vi "IP_POWER1_Off_WebSwitch_Control.vi"() -> ()   [LabVIEW 2011]
doc: "Example of using standard HTTP protocol for recieving a web site (the HTML source)\n\n\nThis example uses the GET command. For general information about the HTTP protocol and other commands go to\nhttp://www.w3.org/Protocols\n\n\nBjornar Svingen\nbjornar.svingen@sintef.no bjornar.svingen@ktv.no"
uses:
  Instance           2 38Saved   IP_POWER_Off_WebSwitch_Control .vi
  Instance           6 38Saved   IP_POWER_Off_WebSwitch_Control .vi
panel:
  out "Begin Time":u32
  out "SW OU2 ON/OFF":bool=TRUE
  out "SW OU1 ON/OFF":bool=TRUE
  out "standard output":string
  out "PING WEBSW IP CMD":string
  out "code 2":i32
  out "Setup WEBSW IP CMD":string
  out "code":i32
  out "WEBSW_SN":string
  out "WEBSW_IP":string
  out "text":string
  out "Setup Status":bool
  out "result string":string
  out "Device SW State":bool[](array[boolean])
  out "Seach the specific string":string[](array[string])
  out "OUT CMD":string[](array[string])
  out "OUT2 CMD":string="/state.xml?relay2State=1"
  out "OUT1 CMD":string="/state.xml?relay1State=1"
  out "HTML source":string
  # "小心它是110V"
  # "2014-10-8"
  # "Web Switch Control"
  # "POWER1 off"
  # "PowerOff"
  # "Command\nhttp://Device IP/state.xml?relay1State=0\nhttp://Device IP/state.xml?relay1State=1\nhttp://Device IP/state.xml?relay2State=0\nhttp://Device IP/state.xml?relay2State=1"
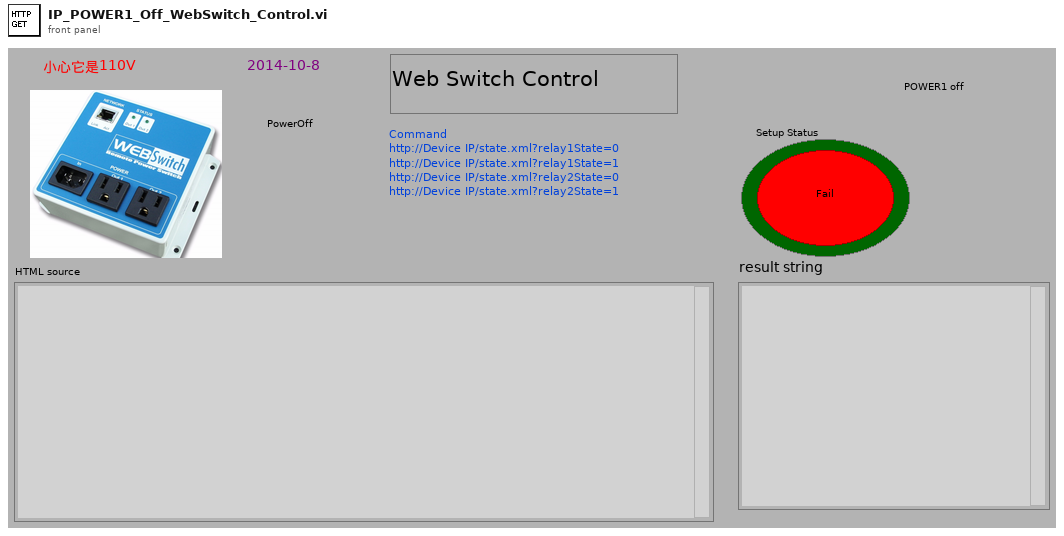
[diagram p1: front panel]
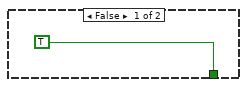
[diagram p5: hidden frame]
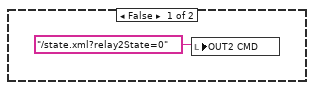
[diagram p7: hidden frame]
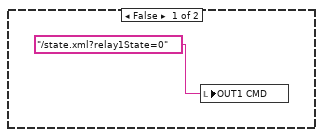
[diagram p8: hidden frame]
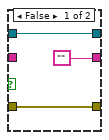
[diagram p9: hidden frame]
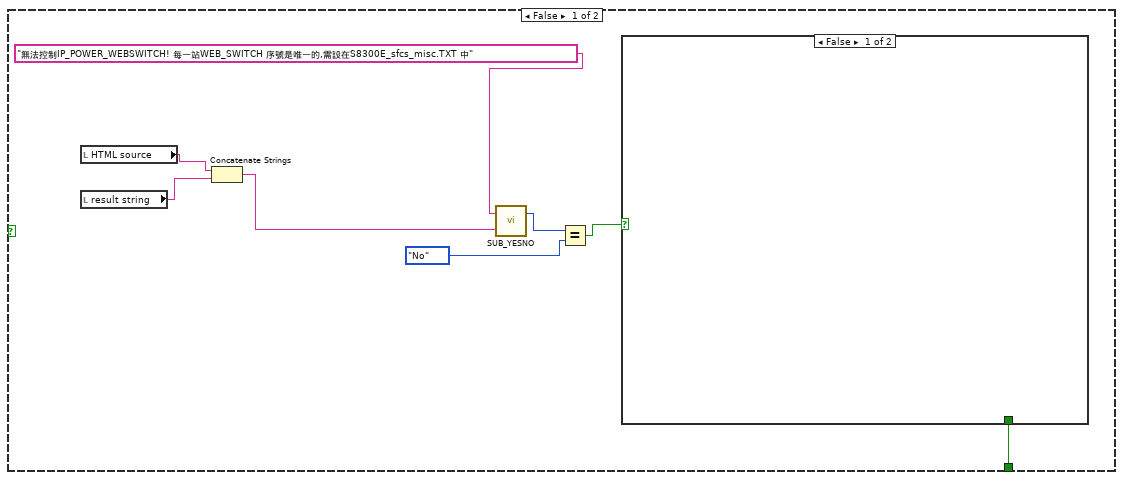
[diagram p10: hidden frame]
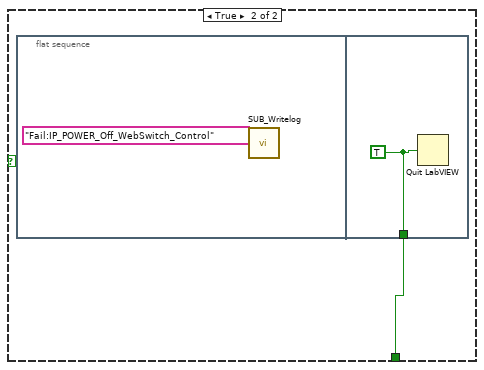
[diagram p11: hidden frame]
diagram:
  n1 = while {
    i -> [w1]
    stop <- w2 stop-if-true
    n2 = flat-sequence {
      tunnel: w1 -> [w4]
      tunnel: [w127] -> w2
      frame #0 {
        n3 = Equal To 0?(x=w4) -> (x = 0?=w3:bool)
        n4 = case shown="True" w3 {
          frame False {
          }
          frame True {
            n5 = Tick Count (ms)() -> (millisecond timer value=→"Begin Time":u32)
          }
        }
      }
      frame #1 {
        w8 = ""
        # "To assign the temporary IP address...\n1. Make sure  WebSwitch TM  and the configuration computer are connected to the same physical\nnetwork.  This will not work through routers or gateways.\n2. Assign the address as follows...\nWindows:\nOpen a Command Prompt (on Windows XP, select START, then RUN, then type “cmd”).\nType...\narp -s {new IP address} {serial number of  WebSwitch TM  }Revision 1.01                           WebSwitch TM    Users Manual\nXytronix Research & Design, Inc.                  page 6\nNote:   IP address format is: xxx.xxx.xxx.xxx\nSerial number format is: ss-ss-ss-ss-ss-ss\nFor example, to set a WebSwitch TM  device (with serial number 00-0C-C8-01-00-01 )  to\n10.10.10.40 the following command would be used.\narp -s 10.10.10.40 00-0c-c8-01-00-01"
        n6 = local write "OUT1 CMD"(w8) -> ()
        n7 = local write "OUT2 CMD"(w8) -> ()
        n8 = local write "result string"(w8) -> ()
        "SW OU1 ON/OFF" <- FALSE ("SW OU1 ON/OFF")
        "SW OU2 ON/OFF" <- FALSE ("SW OU2 ON/OFF")
      }
      frame #2 {
        n9 = call "SUB_SearchFile_inFolder.vi"("Search Filename in Folder"="S8300E_sfcs_misc.TXT") -> ("File Existing True/Flase"=w9:bool)  [unwired: 1 in]
        n10 = case shown="False" w9 {
          frame False {
            n11 = flat-sequence {
              frame #0 {
                n12 = call "Display Message to User2"() -> ()  [unwired: 10 in, 2 out]
              }
              frame #1 {
                n13 = call "SUB_Writelog.vi"("Pass/Fail"="Fail:IP_POWER_Off_WebSwitch_Control") -> ()  [unwired: 2 in]
              }
              frame #2 {
                n14 = Quit LabVIEW(quit? (T)=TRUE) -> ()
              }
            }
          }
          frame True {
          }
        }
      }
      frame #3 {
        n15 = call "SUB_Read_specifFile.vi"("name or relative path"="S8300E_sfcs_misc.TXT") -> ("text"=w19:string)  [unwired: 1 in, 1 out]
        "text" <- w19
        n16 = call "SUB_FindSpecificString.vi"("Find this String"="IP_POWER_WEB_SWITCH_IP=", "String data"=w19) -> ("before \"; \" string"=→"WEBSW_IP":string, "Found"=w17:bool)  [unwired: 2 in]
        n17 = call "SUB_FindSpecificString.vi"("Find this String"="IP_POWER_WEB_SWITCH_SN=", "String data"=w19) -> ("before \"; \" string"=→"WEBSW_SN":string, "Found"=w16:bool)  [unwired: 2 in]
        n18 = And(x=w17, y=w16) -> (x .and. y?=w15:bool)
        n19 = case shown="False" w15 {
          frame False {
            n20 = flat-sequence {
              frame #0 {
                n21 = call "Display Message to User"() -> ()  [unwired: 10 in, 2 out]
              }
              frame #1 {
                n22 = call "SUB_Writelog.vi"("Pass/Fail"="Fail:IP_POWER_Off_WebSwitch_Control") -> ()  [unwired: 2 in]
              }
              frame #2 {
                n23 = Quit LabVIEW(quit? (T)=TRUE) -> ()
              }
            }
          }
          frame True {
          }
        }
      }
      frame #4 {
        n24 = local read "WEBSW_IP"() -> (w26:string)
        n25 = local read "WEBSW_SN"() -> (w29:string)
        n26 = Concatenate Strings("ping -l 102 ", w26, "  -n 1") -> (→"PING WEBSW IP CMD":string)
        n27 = Concatenate Strings("arp -S ", w26, "  ", w29) -> (→"Setup WEBSW IP CMD":string)
      }
      frame #5 {
        n28 = while {
          stop <- w33 stop-if-true
          n29 = flat-sequence {
            tunnel: [w39] -> w32
            tunnel: [w48] -> w33
            tunnel: w32 -> [w45]
            frame #0 {
              n30 = Concatenate Strings("arp -d *" ("string"), "\r") -> (w36:string)
              n31 = call "SUB_run_exeFile_Textv2.vi"("exe filename"=w36) -> ()  [unwired: 1 in, 2 out]
            }
            frame #1 {
              (unwired) "CMD /C"
              n32 = local read "Setup WEBSW IP CMD"() -> (w40:string)
              n33 = Concatenate Strings(w40, "\r") -> (w38:string)
              n34 = call "SUB_run_exeFile_Textv2.vi"("exe filename"=w38) -> ("code"=w37:i32)  [unwired: 1 in, 1 out]
              "code" <- w37
              n35 = Not Equal To 0?(x=w37) -> (x != 0?=w39:bool)
            }
            frame #2 {
              (unwired) "CMD /C"
              n36 = local read "PING WEBSW IP CMD"() -> (w53:string)
              n37 = Concatenate Strings(w53, "\r") -> (w43:string)
              n38 = call "SUB_run_exeFile_Textv2.vi"("exe filename"=w43) -> ("code"=→"code 2":i32, "standard output"=w44:string)  [unwired: 1 in]
              "standard output" <- w44
              n39 = call "SUB_FindSpecificString.vi"("Find this String"="Request timed out", "String data"=w44) -> ("Found"=w50:bool)  [unwired: 2 in, 1 out]
              n40 = call "SUB_FindSpecificString.vi"("Find this String"="unreachable", "String data"=w44) -> ("Found"=w49:bool)  [unwired: 2 in, 1 out]
              n41 = Or(x=w50, y=w49) -> (x .or. y?=w47:bool)
              n42 = Or(x=w47, y=w45) -> (x .or. y?=w46:bool)
              n43 = case shown="True" w46 {
                tunnel: w44 -> [_ w59]
                tunnel: [TRUE w56] -> w48
                frame False {
                }
                frame True {
                  # "cc"
                  n44 = call "SUB_YESNO.vi"("Debug View"=w59, "Status"="無法成功Ping WEB Switch ! WEB SW 序號也要設對於文檔S8300E_sfcs_misc.TXT中!") -> ("yes/no"=w58:enum32{"No Selection", "Yes", "No", "None"})  [unwired: 1 in]
                  n45 = Equal?(x=w58, y=enum32{"No Selection", "Yes", "No", "None"}."No") -> (x = y?=w56:bool)
                  n46 = case shown="True" w56 {
                    frame False {
                    }
                    frame True {
                      n47 = flat-sequence {
                        frame #0 {
                          n48 = call "SUB_Writelog.vi"("Pass/Fail"="Fail:IP_POWER_Off_WebSwitch_Control") -> ()  [unwired: 2 in]
                        }
                        frame #1 {
                          n49 = Quit LabVIEW(quit? (T)=TRUE) -> ()
                        }
                      }
                    }
                  }
                }
              }
            }
          }
        }
      }
      frame #6 {
        n50 = local read "SW OU1 ON/OFF"() -> (w64:bool)
        n51 = local read "SW OU2 ON/OFF"() -> (w63:bool)
        n52 = case shown="True" w64 {
          frame False {
            n53 = local write "OUT1 CMD"("/state.xml?relay1State=0") -> ()
          }
          frame True {
            "OUT1 CMD" <- "/state.xml?relay1State=1"
          }
        }
        n54 = case shown="True" w63 {
          frame False {
            n55 = local write "OUT2 CMD"("/state.xml?relay2State=0") -> ()
          }
          frame True {
            "OUT2 CMD" <- "/state.xml?relay2State=1"
          }
        }
      }
      frame #7 {
        n56 = local read "OUT2 CMD"() -> (w76:string)
        n57 = local read "OUT1 CMD"() -> (w77:string)
        n58 = Build Array(FALSE, FALSE) -> (→"Device SW State":bool[])
        n59 = Build Array("relay1state1", "relay2state1") -> (→"Seach the specific string":string[])
        n60 = Build Array(w77, w76) -> (→"OUT CMD":string[])
      }
      frame #8 {
      }
      frame #9 {
        n61 = for {
          N: 1 -> [_]
          i -> [w89]
          # "Compose the header\n(can include lots of things, see www.w3.org/Protodols)"
          # "The GET method is used to recieve a website.\n\nThe header is composed according to the HTTP 1.1 standard"
          # "Close the connection"
          # "If error code=66, meaning the server\nhas transferred all the data and closed\nthe connection, treat this error as no error."
          # "Read the reply\n(from the GET method)\nin 1024 byte blocks\nand stop on any error."
          # "Write the \"header\"\nto the web site"
          # "Open TCP connection at\nspecifyed web site"
          n62 = local read "WEBSW_IP"() -> (w79:string)
          n63 = TCP Open Connection(address=w79, remote port or service name=u16 80 ("remote port")) -> (connection ID=w85:refnum<k5>, error out=w84:errorcluster)  [unwired: 3 in]
          n64 = local read "OUT CMD"() -> (w96:string[])
          n65 = call <vilib>:"Trim Whitespace.vi"("string"=w79) -> ("trimmed string"=w99:string)  [unwired: 1 in]
          n66 = Index Array(array=w96, index=w89) -> (element=w95:string)
          n67 = call <vilib>:"Trim Whitespace.vi"("string"=w95) -> ("trimmed string"=w103:string)  [unwired: 1 in]
          n68 = local read "Seach the specific string"() -> (w94:string[])
          n69 = Concatenate Strings("GET " ("Command"), w103, " HTTP/1.1" ("Command"), "\r\n" ("string"), "Host: " ("Command"), w99, "\r\n\r\n" ("string")) -> (w97:string)
          n70 = TCP Write(connection ID=w85, data in=w97, error in (no error)=w84) -> (connection ID out=w111:refnum<k5>, error out=w110:errorcluster)  [unwired: 1 in, 1 out]
          n71 = while {
            tunnel: w110 -> [w125]
            tunnel: w111 -> [w124]
            tunnel: [w120] -> w108
            tunnel: [w123] -> w105
            tunnel: [w122] -> w107 mode=indexing
            stop <- w120 stop-if-true
            n72 = TCP Read(connection ID=w124, bytes to read=1024, error in (no error)=w125) -> (connection ID out=w123:refnum<k5>, data out=w122:string, error out=w120:errorcluster)  [unwired: 2 in]
          }
          n73 = Index Array(array=w94, index=w89) -> (element=w91:string)
          n74 = Unbundle By Name(w108) -> ("code"=w113:i32)
          n75 = Concatenate Strings(w107) -> (w106:string)
          n76 = Equal?(x=w113, y=66) -> (x = y?=w112:bool)
          n77 = local read "Device SW State"() -> (w90:bool[])
          n78 = case shown="True" w112 {
            tunnel: ["" w118] -> w93
            tunnel: w106 -> [_ w118]
            tunnel: [w115 errorcluster {"status"=FALSE, "code"=0, "source"=""} ("error in (no error)")] -> w80
            tunnel: w108 -> [w115 _]
            tunnel: w105 -> [w114 w117]
            tunnel: [w114 w117] -> w82
            frame False {
            }
            frame True {
            }
          }
          "HTML source" <- w93
          n79 = TCP Close Connection(connection ID=w82, abort (F)=TRUE, error in (no error)=w80) -> (error out=w83:errorcluster)  [unwired: 1 out]
          n80 = call <vilib>:"Simple Error Handler.vi"("error in (no error)"=w83) -> ()  [unwired: 4 in, 5 out]
          n81 = call "SUB_OUT_String_token.vi"("input string"=w93) -> ("result string"=w92:string)  [unwired: 2 in]
          "result string" <- w92
          n82 = call "SUB_FindSpecificString.vi"("Find this String"=w91, "String data"=w92) -> ("Found"=w88:bool)  [unwired: 2 in, 1 out]
          n83 = Replace Array Subset(array=w90, new element=w88, index=w89) -> (w87:bool[])
          n84 = local write "Device SW State"(w87) -> ()
        }
      }
      frame #10 {
        n85 = local read "Device SW State"() -> (w134:bool[])
        n86 = local read "SW OU1 ON/OFF"() -> (w130:bool)
        n87 = Index Array(array=w134) -> (element #1=w133:bool, element #2=w132:bool)  [unwired: 2 in]
        n88 = local read "SW OU2 ON/OFF"() -> (w129:bool)
        n89 = Equal?(x=w130, y=w133) -> (x = y?=w131:bool)
        n90 = Equal?(x=w129, y=w132) -> ()  [unwired: 1 out]
        n91 = And(x=w131, y=TRUE) -> (x .and. y?=w128:bool)
        "Setup Status" <- w128
        n92 = case shown="True" w128 {
          tunnel: [w135 w146] -> w127
          frame False {
            n93 = local read "HTML source"() -> (w141:string)
            n94 = local read "result string"() -> (w140:string)
            n95 = Concatenate Strings(w141, w140) -> (w139:string)
            n96 = call "SUB_YESNO.vi"("Debug View"=w139, "Status"="無法控制IP_POWER_WEBSWITCH! 每一站WEB_SWITCH 序號是唯一的,需設在S8300E_sfcs_misc.TXT 中") -> ("yes/no"=w138:enum32{"No Selection", "Yes", "No", "None"})  [unwired: 1 in]
            n97 = Equal?(x=w138, y=enum32{"No Selection", "Yes", "No", "None"}."No") -> (x = y?=w136:bool)
            n98 = case shown="False" w136 {
              tunnel: [_ w143] -> w135
              frame False {
              }
              frame True {
                n99 = flat-sequence {
                  tunnel: [w145] -> w143
                  frame #0 {
                    n100 = call "SUB_Writelog.vi"("Pass/Fail"="Fail:IP_POWER_Off_WebSwitch_Control") -> ()  [unwired: 2 in]
                  }
                  frame #1 {
                    w145 = TRUE ("quit? (T)")
                    n101 = Quit LabVIEW(quit? (T)=w145) -> ()
                  }
                }
              }
            }
          }
          frame True {
            n102 = flat-sequence {
              tunnel: [w154] -> w146
              frame #0 {
                n103 = local read "Begin Time"() -> (w152:u32)
                n104 = Tick Count (ms)() -> (millisecond timer value=w148:u32)
                n105 = call "SUB_CAL_TESTTIME.vi"("Test Item name"="IP_POWER_Off_WebSwitch_Control", "Stop tick time"=w148, "Start tick time"=w152) -> ("Test Time output"=w150:string)  [unwired: 2 in]
                n106 = Concatenate Strings("Pass:IP_POWER_Off_WebSwitch_Control", w150) -> (w149:string)
                n107 = call "SUB_Writelog.vi"("Pass/Fail"=w149) -> ()  [unwired: 2 in]
              }
              frame #1 {
                n108 = Wait (ms)(milliseconds to wait=u32 500) -> ()  [unwired: 1 out]
              }
              frame #2 {
                w154 = TRUE ("quit? (T)")
                n109 = Quit LabVIEW(quit? (T)=w154) -> ()
              }
            }
          }
        }
      }
    }
  }
